vi "Configure Power Measurement Filter.vi"(7 "Bandwidth (100kHz)":dbl=100000.0 format="%#.9p", 8 "error in (no error)":errorcluster, 9 "Filter Type (Gauss)":i32(ring) items=["Gauss", "Bandpass", "WCDMA", "CDMA", "TD-SCDMA"], 10 "Instance (1)":i32=1 format="%.0g", 11 "VISA resource name":refnum<visa-resource-name>) -> (0 "error out":errorcluster, 3 "VISA resource name out":refnum<visa-resource-name>)   [LabVIEW 2020, in "Rohde&Schwarz CMXP GPRF.lvlib"]
doc: "Configures power measurement filter type and bandwidth.\n\nAttributes:\nRSCMXPGPRF_ATTR_POWER_MEASUREMENT_FILTER_TYPE\nRSCMXPGPRF_ATTR_POWER_MEASUREMENT_GAUSS_BANDWIDTH\nRSCMXPGPRF_ATTR_POWER_MEASUREMENT_BANDPASS_BANDWIDTH\n\nRemote-control commands:\nCONFigure:GPRF:MEAS<i>:POWer:FILTer:TYPE\nCONFigure:GPRF:MEAS<i>:POWer:FILTer:GAUSs:BWIDth\nCONFigure:GPRF:MEAS<i>:POWer:FILTer:BANDpass:BWIDth"
uses:
  <instrlib>/Rohde&Schwarz CMXP GPRF/Rohde&Schwarz CMXP GPRF.lvlib
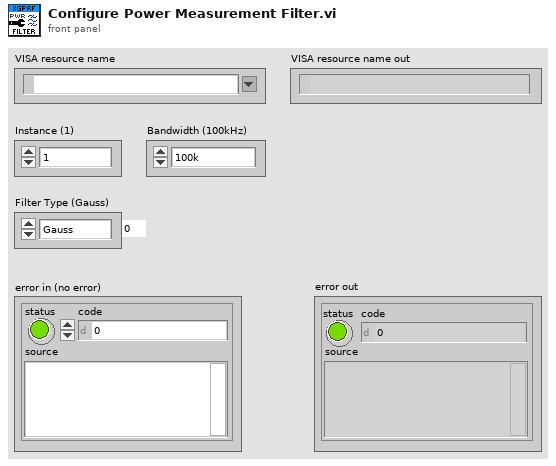
[diagram p1: front panel]
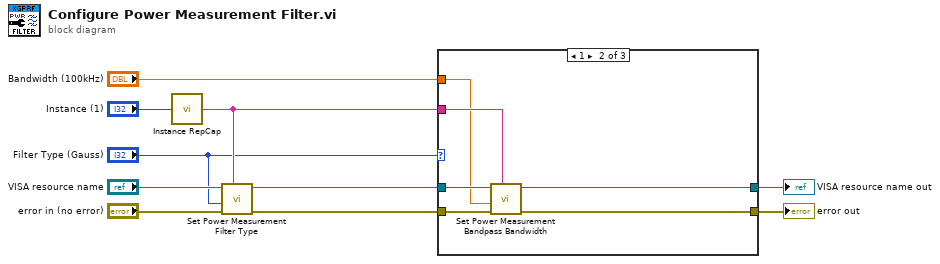
[diagram p0: block diagram]
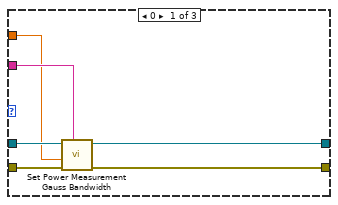
[diagram p2: hidden frame]
diagram:
  n1 = call <instrlib>:"Instance RepCap.vi"("Instance in"="Instance (1)") -> ("Instance out"=w4:string)
  n2 = call "Set Power Measurement Filter Type"("Repeated Capabilities"=w4, "error in (no error)"="error in (no error)", "Power Measurement Filter Type (0 - Gauss)"="Filter Type (Gauss)", "instrument handle"="VISA resource name") -> ("error out"=w8:errorcluster, "instrument handle out"=w5:refnum<visa-resource-name>)  [unwired: 6 in]
  n3 = case shown="1" "Filter Type (Gauss)" {
    tunnel: w8 -> [w16 w22 w24]
    tunnel: [w13 w19 w24] -> w7
    tunnel: [w12 w18 w23] -> w6
    tunnel: w5 -> [w15 w21 w23]
    tunnel: w4 -> [w14 w20 _]
    tunnel: "Bandwidth (100kHz)" -> [w11 w17 _]
    frame 0 {
      n4 = call "Set Power Measurement Gauss Bandwidth"("Repeated Capabilities"=w14, "error in (no error)"=w16, "Power Measurement Gauss Bandwidth (0.0)"=w11, "instrument handle"=w15) -> ("error out"=w13:errorcluster, "instrument handle out"=w12:refnum<visa-resource-name>)  [unwired: 6 in]
    }
    frame 1 {
      n5 = call "Set Power Measurement Bandpass Bandwidth"("Repeated Capabilities"=w20, "error in (no error)"=w22, "Power Measurement Bandpass Bandwidth (0.0)"=w17, "instrument handle"=w21) -> ("error out"=w19:errorcluster, "instrument handle out"=w18:refnum<visa-resource-name>)  [unwired: 6 in]
    }
    frame 2, Default {
    }
  }
  "error out" <- w7
  "VISA resource name out" <- w6
